vi "Get Test Log.vi"(11 "Model in":refnum<class "Model.lvclass">) -> (2 "TestLog":refnum<class "Test Log.lvclass">, 3 "Model out":refnum<class "Model.lvclass">)   [LabVIEW 2015, in "Model.lvclass"]
uses:
  Model.lvclass
  Test Log/Test Log/Test Log.lvclass
  Model.lvclass/Model.ctl
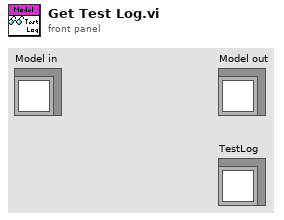
[diagram p1: front panel]
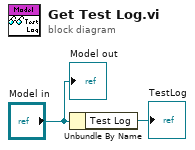
[diagram p0: block diagram]
diagram:
  n1 = Unbundle By Name("Model in") -> ("Test Log"=→"TestLog":refnum<class "Test Log.lvclass">)
  "Model out" <- "Model in"
